vi "PRN Generation_Station1.vi"(0 "Part PRN QR":path, 3 "error in (no error)":errorcluster, 4 "Cluster":T2) -> (6 "QR Code":string, 7 "PRN to Print":string, 10 "error out":errorcluster)   [LabVIEW 2017]
uses:
  <vilib>/addons/database/Connection.llb/Conn ObjectReference.ctl
  <vilib>/addons/database/NI_Database_API.lvlib
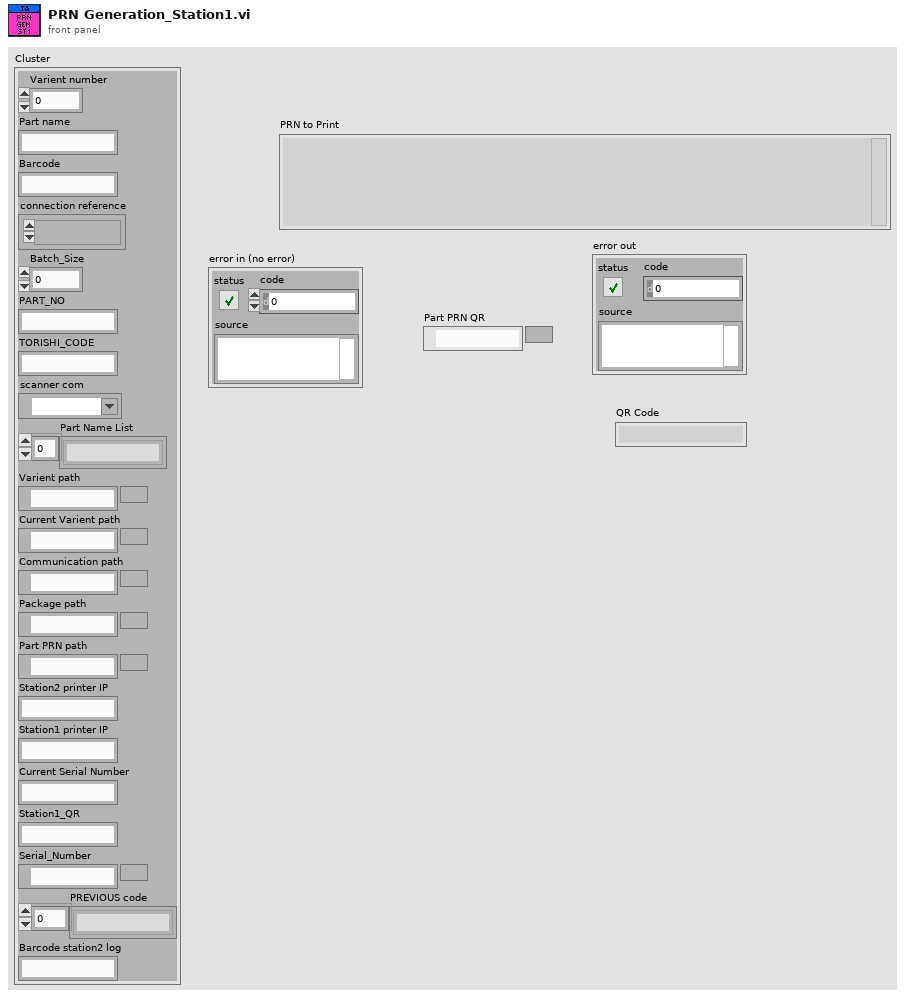
[diagram p1: front panel]
types:
  T1 = typedef "NI_Database_API.lvlib/Conn ObjectReference.ctl" = refnum<k1>
  T2 = cluster{"Varient number":u16, "Part name":string, "Barcode":string, "connection reference":T1, "Batch_Size":u16, "PART_NO":string, "TORISHI_CODE":string, "scanner com":refnum<visa-resource-name>, "Part Name List":string[], "Varient path":path, "Current Varient path":path, "Communication path":path, "Package path":path, "Part PRN path":path, "Station2 printer IP":string, "Station1 printer IP":string, "Current Serial Number":string, "Station1_QR":string, "Serial_Number":path, "PREVIOUS code":string[], "Barcode station2 log":string}
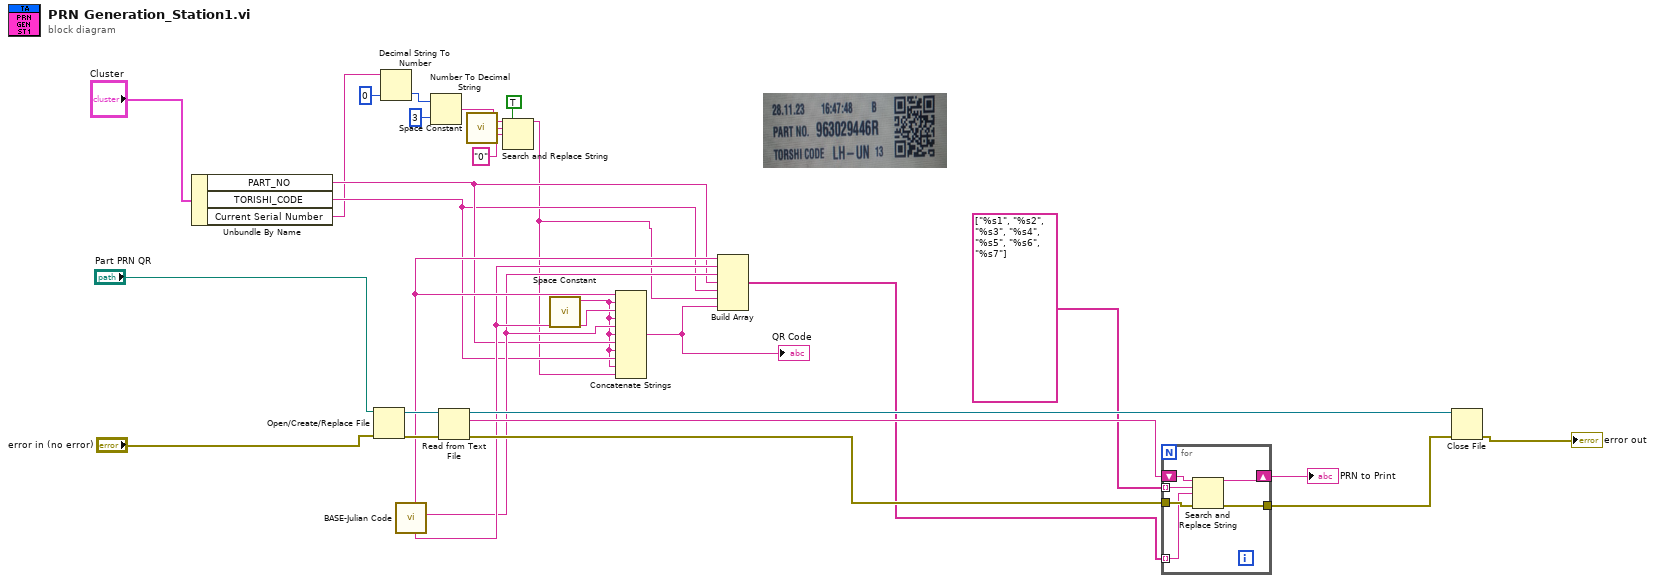
[diagram p0: block diagram]
diagram:
  n1 = Unbundle By Name("Cluster") -> ("PART_NO"=w14:string, "TORISHI_CODE"=w13:string, "Current Serial Number"=w2:string)
  n2 = Open/Create/Replace File(file path (use dialog)="Part PRN QR", error in="error in (no error)") -> (refnum out=w26:refnum<file>, error out=w27:errorcluster)  [unwired: 4 in, 1 out]
  n3 = Decimal String To Number(string=w2, default (0L)=0 ("default (0 I32)")) -> (number=w8:i32)  [unwired: 1 in, 1 out]
  n4 = call "BASE-Julian Code.vi"() -> ("Shift"=w15:string, "Long time with :"=w16:string, "Long date with /"=w17:string)  [unwired: 6 in, 3 out]
  n5 = Number To Decimal String(number=w8, width (-)=i16 3) -> (decimal integer string=w6:string)
  n6 = Read from Text File(file (use dialog)=w26, error in=w27) -> (refnum out=w28:refnum<file>, text=w24:string, error out=w22:errorcluster)  [unwired: 2 in, 1 out]
  n7 = call <vilib>:"Space Constant.vi"() -> ("String"=w5:string)
  n8 = Search and Replace String(replace all?=TRUE ("replace all? (F)"), input string=w6, search string=w5, replace string="0" ("replace string (\"\")")) -> (result string=w1:string)  [unwired: 4 in, 3 out]
  n9 = call <vilib>:"Space Constant.vi"() -> ("String"=w12:string)
  n10 = Concatenate Strings(w17, w12, w16, w12, w15, w12, w14, w12, w13, w12, w1) -> (w10:string)
  "QR Code" <- w10
  n11 = Build Array(w17, w16, w15, w14, w13, w1, w10) -> (w11:string[])
  n12 = for {
    shift-right: [w34] -> w23
    shift-left: w24 -> [w35]
    tunnel: w22 -> [w33]
    tunnel: [w32] -> w21
    tunnel: string[] ["%s1", "%s2", "%s3", "%s4", "%s5", "%s6", "%s7"] -> [w31] mode=indexing
    tunnel: w11 -> [w30] mode=indexing
    n13 = Search and Replace String(input string=w35, search string=w31, replace string=w30, error in=w33) -> (result string=w34:string, error out=w32:errorcluster)  [unwired: 4 in, 2 out]
  }
  "PRN to Print" <- w23
  n14 = Close File(refnum=w28, error in=w21) -> (error out=→"error out":errorcluster)  [unwired: 1 out]
